vi "Default Config--constant.vi"() -> (3 "Default Config":T1)   [LabVIEW 2023, in "VI Properties Editor.lvlib"]
uses:
  VI Properties Editor.lvlib
  CTLs/Config.ctl
  <vilib>/Utility/sysdir.llb/System Directory Type.ctl
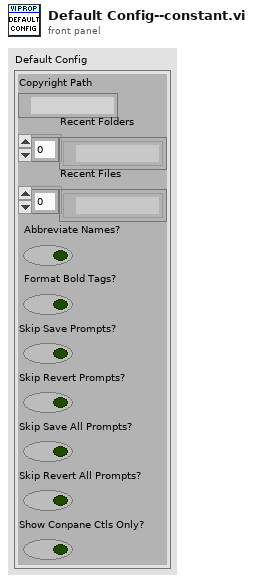
[diagram p1: front panel]
types:
  T1 = typedef "VI Properties Editor.lvlib/Config.ctl" = cluster{"Copyright Path":path, "Recent Folders":path[], "Recent Files":path[], "Abbreviate Names?":bool, "Format Bold Tags?":bool, "Skip Save Prompts?":bool, "Skip Revert Prompts?":bool, "Skip Save All Prompts?":bool, "Skip Revert All Prompts?":bool, "Show Conpane Ctls Only?":bool}
  T2 = typedef "System Directory Type.ctl" = i32
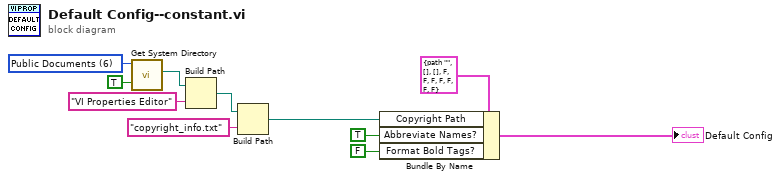
[diagram p0: block diagram]
diagram:
  w6 = T2 6 items=["User Home"=0, "User Desktop"=1, "User Documents"=2, "User Application Data"=3, "User Preferences"=4, "User Temporary"=5, "Public Documents"=6, "Public Application Data"=7, "Public Preferences"=8, "Public Cache"=13, "System Core Libraries"=9, "System Installed Libraries"=10, "Application Files"=11, "Boot Volume Root"=12] ("system directory type")
  n1 = call <vilib>:"Get System Directory.vi"("create directory if not found? (F)"=TRUE, "system directory type"=w6) -> ("system directory"=w8:path)  [unwired: 9 in]
  n2 = Build Path(base path=w8, name or relative path="VI Properties Editor") -> (appended path=w2:path)
  n3 = Build Path(base path=w2, name or relative path="copyright_info.txt") -> (appended path=w1:path)
  n4 = Bundle By Name(cluster=T1 {"Copyright Path"=path "", "Recent Folders"=[], "Recent Files"=[], "Abbreviate Names?"=FALSE, "Format Bold Tags?"=FALSE, "Skip Save Prompts?"=FALSE, "Skip Revert Prompts?"=FALSE, "Skip Save All Prompts?"=FALSE, "Skip Revert All Prompts?"=FALSE, "Show Conpane Ctls Only?"=FALSE} ("Config"), "Copyright Path"=w1, "Abbreviate Names?"=TRUE, "Format Bold Tags?"=FALSE ("View Formatted Bold")) -> (→"Default Config":T1)
